vi "OutputClimber.vi"   [LabVIEW 2023]
doc: "This VI sends commands to the arm subsystem."
uses:
  GRNF_CTREMotor.vi
  GlobalClimber.vi
types:
  T1 = enum16{"No Changed Output", "New Normal Output", "New Testing Output"}
  T2 = typedef "WPI_MotorControlDeviceRef.ctl" = cluster{"DeviceStatus":errorcluster, "Type":T3, "PWM":cluster{"PWM Channel":T4, "DeadBand":T5}, "CAN":cluster{"Device Number":u8, "SetOutput VI Ref":variant, "GetOutput VI Ref":variant, "Enable VI Ref":variant, "Disable VI Ref":variant, "Data":variant}, "Invert":bool, "DIO PWM":cluster{"PWM \"Enable\" Channel":T4, "DIOChannel":T6, "PWM Rate":dbl}}
  T3 = typedef "WPI_MotorControlType.ctl" = enum16{"PWM", "CAN", "DIO PWM"}
  T4 = typedef "FPGA_DIOPWMChannel.ctl" = enum8{"PWM 0", "PWM 1", "PWM 2", "PWM 3", "PWM 4", "PWM 5", "PWM 6", "PWM 7", "PWM 8", "PWM 9", "PWM MXP 0", "PWM MXP 1", "PWM MXP 2", "PWM MXP 3", "PWM MXP 4", "PWM MXP 5", "PWM MXP 6", "PWM MXP 7", "PWM MXP 8", "PWM MXP 9", "Invalid"}
  T5 = typedef "WPI_PWMDeadband.ctl" = cluster{"Name":string, "maxPositivePwm":i32, "minPositivePwm":i32, "centerPwm":i32, "maxNegativePwm":i32, "minNegativePwm":i32, "angularRange":u16}
  T6 = typedef "FPGA_DIOChannel.ctl" = enum8{"DIO 0", "DIO 1", "DIO 2", "DIO 3", "DIO 4", "DIO 5", "DIO 6", "DIO 7", "DIO 8", "DIO 9", "DIO MXP 0", "DIO MXP 1", "DIO MXP 2", "DIO MXP 3", "DIO MXP 4", "DIO MXP 5", "DIO MXP 6", "DIO MXP 7", "DIO MXP 8", "DIO MXP 9", "DIO MXP 10", "DIO MXP 11", "DIO MXP 12", "DIO MXP 13", "DIO MXP 14", "DIO MXP 15", "SPI Port CS1", "SPI Port CS2", "SPI Port CS3", "SPI Port MISO", "SPI Port MOSI", "Invalid"}
  T7 = typedef "WPI_SolenoidDevRef.ctl" = cluster{"DevStatus":errorcluster, "Pneumatics Control Module":u8, "Forward Solenoid Channel":T8, "Reverse Solenoid Channel":T8}
  T8 = typedef "WPI_SolenoidChannel.ctl" = enum8{"Solenoid 0", "Solenoid 1", "Solenoid 2", "Solenoid 3", "Solenoid 4", "Solenoid 5", "Solenoid 6", "Solenoid 7", "Solenoid 8", "Solenoid 9", "Solenoid 10", "Solenoid 11", "Solenoid 12", "Solenoid 13", "Solenoid 14", "Solenoid 15", "Invalid"}
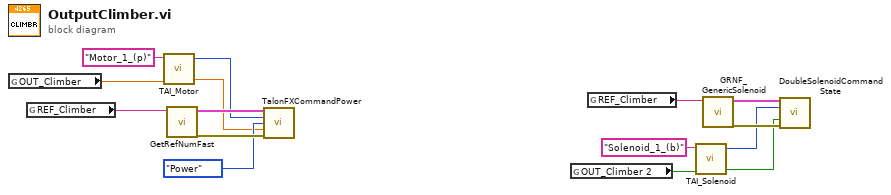
[diagram p0: block diagram]
diagram:
  n1 = global read "GlobalClimber.vi" "OUT_Climber"() -> (w4:dbl)
  n2 = global read "GlobalClimber.vi" "REF_Climber"() -> (w3:string)
  n3 = call "TAI_Motor.vi"("Normal Output"=w4, "Actuator Name"="Motor_1_(p)") -> ("Interlocked Output"=w10:dbl, "Testing Mode"=w11:T1)  [unwired: 3 in]
  n4 = call-poly "GetRefNumFast.vi"("RefNum Name"=w3) -> ("Error"=w13:errorcluster, "Device Reference"=w14:T2)  [unwired: 5 in]
  n5 = call "TalonFXCommandPower.vi"("Device Reference (in)"=w14, "Output Mode"=w11, "Control Mode"=enum16{"Safety", "Power"}."Power", "Power or Testing Power"=w10, "Error (in)"=w13) -> ()  [unwired: 11 in]
  n6 = global read "GlobalClimber.vi" "OUT_Climber 2"() -> (w1:bool)
  n7 = global read "GlobalClimber.vi" "REF_Climber"() -> (w2:string)
  n8 = call "TAI_Solenoid.vi"("Normal Output"=w1, "Actuator Name"="Solenoid_1_(b)") -> ("Interlocked Output"=w5:bool, "Output Mode"=w6:T1)  [unwired: 3 in]
  n9 = call "GRNF_GenericSolenoid.vi"("RefNum Name"=w2) -> ("Error"=w7:errorcluster, "Device Reference"=w8:T7)  [unwired: 5 in]
  n10 = call "DoubleSolenoidCommandState.vi"("Device Reference (in)"=w8, "Output Mode"=w6, "State [True, False]"=w5, "Error (in)"=w7) -> ()  [unwired: 12 in]
